vi "PicoScope6000IsReady.vi"(8 "error in (no error)":errorcluster, 11 "handle in":i16) -> (0 "error out":errorcluster, 3 "handle out":i16, 6 "ready":i16)   [LabVIEW 2009]
doc: "Calls IsReady function."
uses:
  ps6000.dll
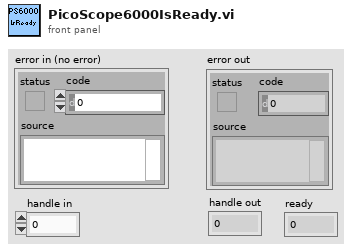
[diagram p1: front panel]
types:
  T1 = cluster{"status":bool, "code":u32, "source":string}
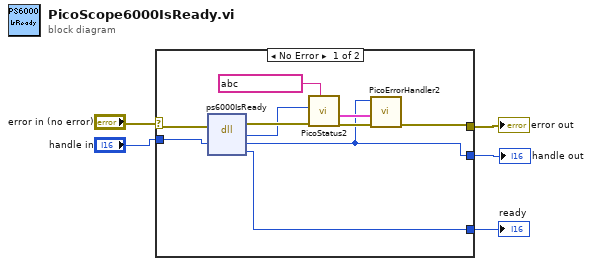
[diagram p0: block diagram]
diagram:
  n1 = case shown="No Error" "error in (no error)" {
    selector: "error in (no error)" -> [w15 w16]
    tunnel: "handle in" -> [w14 w17]
    tunnel: [w8 w17] -> w5
    tunnel: [w10 w16] -> w4
    tunnel: [w7 _] -> w3
    frame #0 {
      n2 = dll-call lib="PS6000.dll" fn="ps6000IsReady" ("ps3000.dll:_ps3000_open_unit@0")(error in=w15, "handle"=w14) -> (error out=w11:errorcluster, "status"=w9:u32, "handle"=w8:i16, "ready"=w7:i16)  [unwired: 3 in, 1 out]
      n3 = call "PicoStatus2.vi"("PICO source"=string ? ("source"), "Error in"=w11, "PICO STATUS"=w9) -> ("error out"=w13:errorcluster, "PICO_STATUS out"=w12:T1)  [unwired: 5 in]
      n4 = call "PicoErrorHandler2.vi"("error in (no error)"=w13, "PICO_STATUS in"=w12, "handle In"=w8) -> ("error out"=w10:errorcluster)  [unwired: 8 in]
    }
    frame #1 {
    }
  }
  "error out" <- w4
  "handle out" <- w5
  "ready" <- w3
